vi "C2P_zero.vi"(0 "r * e^(i*theta)":cdb[](array[numeric]) format="%0.2f") -> (1 "amplitude":dbl[](array[numeric]) format="%0.2f", 2 "phase":dbl[](array[numeric]) format="%0.2f")   [LabVIEW 2017, in "NI_PtbyPt.lvlib"]
doc: "Truncates the extremely small complex value to zero, both amplitude and phase."
uses:
  <vilib>/ptbypt/NI_PtbyPt.lvlib
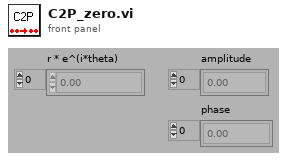
[diagram p1: front panel]
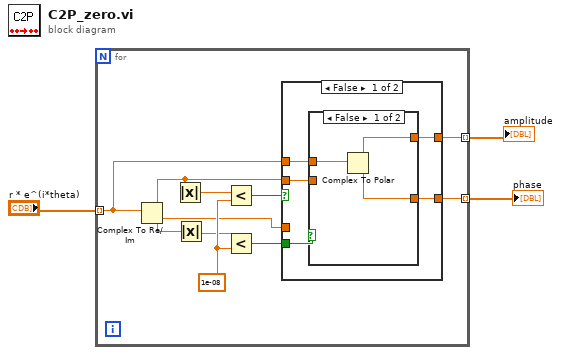
[diagram p0: block diagram]
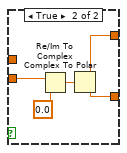
[diagram p2: hidden frame]
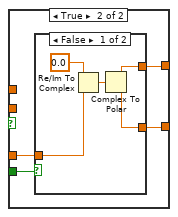
[diagram p3: hidden frame]
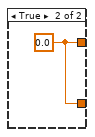
[diagram p4: hidden frame]
diagram:
  n1 = for {
    tunnel: "r * e^(i*theta)" -> [w10] mode=indexing
    tunnel: [w8] -> w1 mode=indexing
    tunnel: [w7] -> w2 mode=indexing
    w13 = 1e-08
    n2 = Complex To Re/Im(x + iy=w10) -> (x=w4:dbl, y=w9:dbl)
    n3 = Absolute Value(x=w4) -> (abs(x)=w5:dbl)
    n4 = Absolute Value(x=w9) -> (abs(x)=w6:dbl)
    n5 = Less?(x=w5, y=w13) -> (x < y?=w12:bool)
    n6 = Less?(x=w6, y=w13) -> (x < y?=w11:bool)
    n7 = case shown="False" w12 {
      tunnel: w11 -> [w18 w30]
      tunnel: w10 -> [w17 _]
      tunnel: [w16 w29] -> w7
      tunnel: [w15 w28] -> w8
      tunnel: w9 -> [_ w27]
      tunnel: w4 -> [w14 _]
      frame False {
        n8 = case shown="False" w18 {
          tunnel: w17 -> [w21 _]
          tunnel: [w20 w23] -> w16
          tunnel: [w19 w22] -> w15
          tunnel: w14 -> [_ w24]
          frame False {
            n9 = Complex To Polar(r * e^(i*theta)=w21) -> (r=w20:dbl, theta=w19:dbl)
          }
          frame True {
            n10 = Re/Im To Complex(1:0.0, 2:w24) -> (0:w26:cdb)
            n11 = Complex To Polar(r * e^(i*theta)=w26) -> (r=w23:dbl, theta=w22:dbl)
          }
        }
      }
      frame True {
        n12 = case shown="False" w30 {
          tunnel: [w32 w36] -> w29
          tunnel: [w31 w36] -> w28
          tunnel: w27 -> [w34 _]
          frame False {
            n13 = Re/Im To Complex(1:w34, 2:0.0) -> (0:w33:cdb)
            n14 = Complex To Polar(r * e^(i*theta)=w33) -> (r=w32:dbl, theta=w31:dbl)
          }
          frame True {
            w36 = 0.0
          }
        }
      }
    }
  }
  "amplitude" <- w2
  "phase" <- w1
